vi "subGetBuildSpecRefsFromProject.vi"(11 "Project refs":refnum<vi>[](array[refnum])) -> (3 "Spec and project refs":map{string, T1}(c390))   [LabVIEW 2020, in "SolutionBuilder.lvlib" / "SolutionBuilder.lvclass"]
uses:
  SolutionBuilder.lvclass
  Private/SpecAndProject.ctl
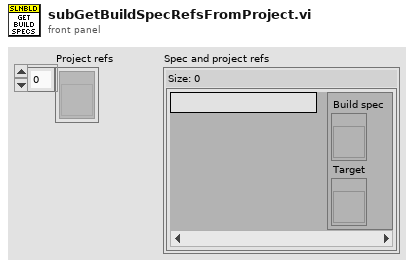
[diagram p1: front panel]
types:
  T1 = typedef "SolutionBuilder.lvlib/SolutionBuilder.lvclass/SpecAndProject.ctl" = cluster{"Build spec":refnum<vi>, "Target":refnum<vi>}
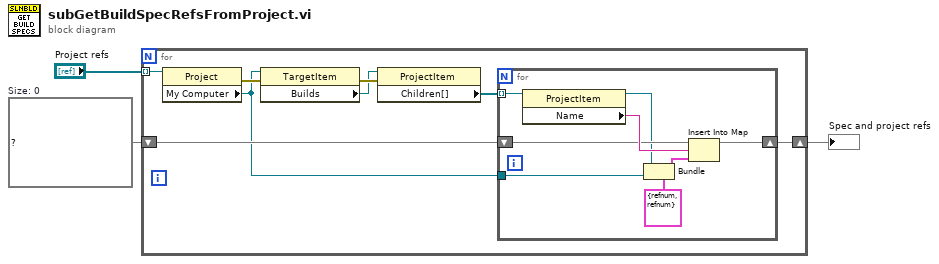
[diagram p0: block diagram]
diagram:
  w2 = map{string, T1} {}  # Size: 0
  n1 = for {
    tunnel: "Project refs" -> [w5] mode=indexing
    shift-right: [w8] -> w1
    shift-left: w2 -> [w7]
    n2 = property class="Project"(reference=w5) -> (error out=w10:errorcluster, "My Computer"=w4:refnum<vi>)  [unwired: 1 in, 1 out]
    n3 = property class="TargetItem"(reference=w4, error in=w10) -> (error out=w11:errorcluster, "Builds"=w6:refnum<vi>)  [unwired: 1 out]
    n4 = property class="ProjectItem"(reference=w6, error in=w11) -> ("Children[]"=w9:refnum<vi>[])  [unwired: 2 out]
    n5 = for {
      tunnel: w9 -> [w19] mode=indexing
      shift-right: [w17] -> w8
      shift-left: w7 -> [w16]
      tunnel: w4 -> [w14]
      n6 = property class="ProjectItem"(reference=w19) -> (reference out=w15:refnum<vi>, "Name"=w18:string)  [unwired: 1 in, 1 out]
      n7 = Bundle(cluster=T1 {"Build spec"=refnum, "Target"=refnum} ("Cluster"), "Build spec"=w15, "Target"=w14) -> (w13:T1)
      n8 = Insert Into Map(map in=w16, key=w18, value=w13) -> (map out=w17:map{string, T1})  [unwired: 2 out]
    }
  }
  "Spec and project refs" <- w1
